vi "StartupGISPollProcess.vi"(8 "error in (no error)":errorcluster, 10 "GIS Printer":refnum<class "GIS Printer.lvclass">, 11 "TopLevel in":refnum<class "TopLevel.lvclass">) -> (0 "error out":errorcluster)   [LabVIEW 2022 SP3, in "GIS Printer.lvclass"]
uses:
  GIS Printer.lvclass
  TopLevel/TopLevel.lvclass
  GIS Poll Process.vi
  GIS Head Poll Process.vi
panel:
  out "Array 2":bool[](array[boolean])
  out "Array":bool[](array[boolean])
  out "timed out?":bool
  out "sync from process?":bool
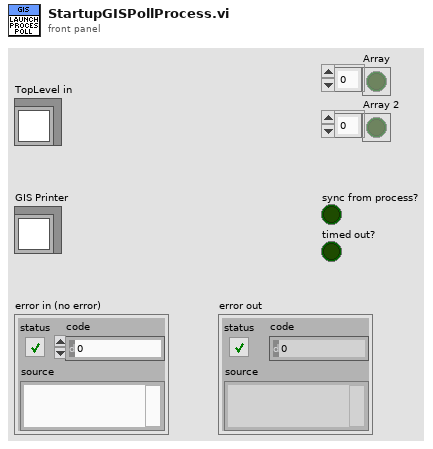
[diagram p1: front panel]
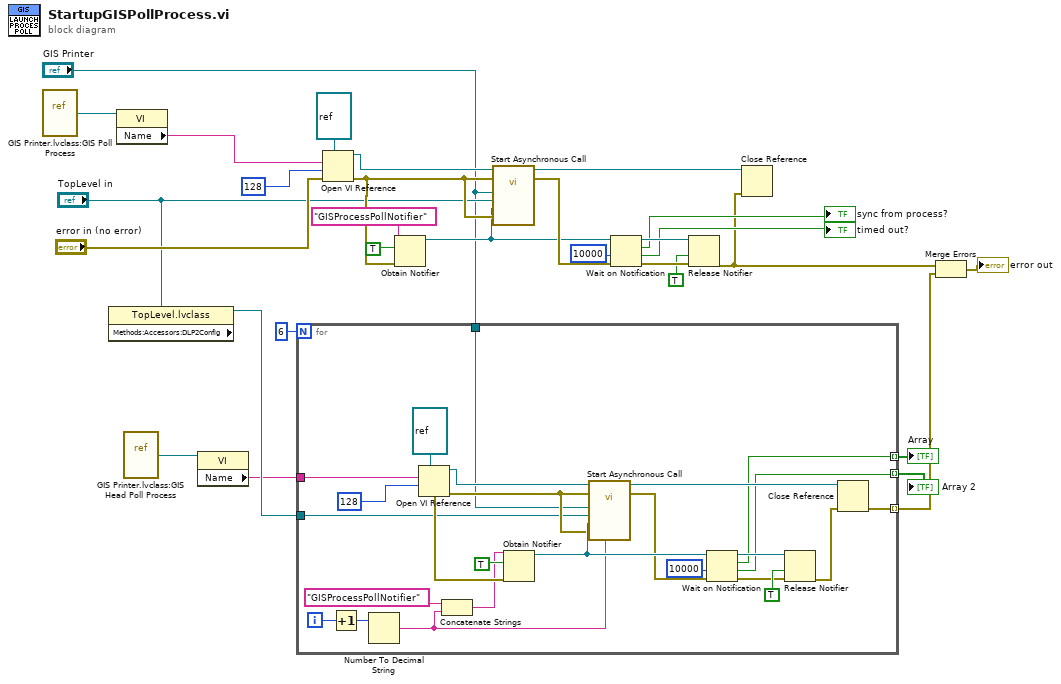
[diagram p0: block diagram]
diagram:
  n1 = vi-ref "GIS Printer.lvclass:GIS Poll Process.vi"() -> (w23:refnum<vi>)
  n2 = property class="TopLevel.lvclass" props=["Methods:Accessors:DLP2Config"](reference="TopLevel in") -> (reference out=w8:refnum<class "TopLevel.lvclass">)  [unwired: 1 in, 2 out]
  n3 = property class="VI"(reference=w23) -> ("Name"=w24:string)  [unwired: 1 in, 2 out]
  n4 = vi-ref "GIS Printer.lvclass:GIS Head Poll Process.vi"() -> (w9:refnum<vi>)
  n5 = property class="VI"(reference=w9) -> ("Name"=w6:string)  [unwired: 1 in, 2 out]
  n6 = for {
    N: 6 -> [_]
    tunnel: w8 -> [w37]
    tunnel: "GIS Printer" -> [w36]
    tunnel: w6 -> [w35]
    tunnel: [w34] -> w2 mode=indexing
    tunnel: [w33] -> w1 mode=indexing
    tunnel: [w31] -> w3 mode=indexing
    i -> [w40]
    n7 = Increment(x=w40) -> (x+1=w32:i32)
    n8 = Number To Decimal String(number=w32) -> (decimal integer string=w30:string)  [unwired: 1 in]
    n9 = Open VI Reference(type specifier VI Refnum (for type only)=refnum<vi> refnum, vi path=w35, options=128) -> (vi reference=w43:refnum<vi>, error out=w46:errorcluster)  [unwired: 3 in]
    n10 = Concatenate Strings("GISProcessPollNotifier" ("name (unnamed)"), w30) -> (w38:string)
    n11 = Obtain Notifier(name (unnamed)=w38, notification data type=TRUE, error in (no error)=w46) -> (notifier out=w53:refnum<notifier>)  [unwired: 1 in, 2 out]
    n12 = call-by-ref "Start Asynchronous Call"(reference=w43, error in=w46, "HeadNo"=w30, 8:"error in (no error)"=w46, "notifierSync"=w53, "TopLevel"=w37, "GIS Printer in"=w36) -> (reference out=w42:refnum<vi>, error out=w51:errorcluster)  [unwired: 5 in, 2 out]
    n13 = Wait on Notification(notifier=w53, timeout in ms (-1)=10000, error in (no error)=w51) -> (notifier out=w49:refnum<notifier>, notification=w34:bool, timed out?=w33:bool, error out=w48:errorcluster)  [unwired: 1 in]
    n14 = Release Notifier(notifier=w49, force destroy? (F)=TRUE, error in (no error)=w48) -> (error out=w52:errorcluster)  [unwired: 2 out]
    n15 = Close Reference(reference=w42, error in (no error)=w52) -> (error out=w31:errorcluster)
  }
  "Array" <- w2
  "Array 2" <- w1
  n16 = Open VI Reference(type specifier VI Refnum (for type only)=refnum<vi> refnum, vi path=w24, options=128, error in (no error)="error in (no error)") -> (vi reference=w26:refnum<vi>, error out=w20:errorcluster)  [unwired: 2 in]
  n17 = Obtain Notifier(name (unnamed)="GISProcessPollNotifier", notification data type=TRUE, error in (no error)=w20) -> (notifier out=w11:refnum<notifier>)  [unwired: 1 in, 2 out]
  n18 = call-by-ref "Start Asynchronous Call"(reference=w26, error in=w20, 8:"error in (no error)"=w20, "notifierSync"=w11, "TopLevel"="TopLevel in", "GIS Printer in"="GIS Printer") -> (reference out=w27:refnum<vi>, error out=w13:errorcluster)  [unwired: 6 in, 2 out]
  n19 = Wait on Notification(notifier=w11, timeout in ms (-1)=10000, error in (no error)=w13) -> (notifier out=w17:refnum<notifier>, notification=→"sync from process?":bool, timed out?=→"timed out?":bool, error out=w18:errorcluster)  [unwired: 1 in]
  n20 = Release Notifier(notifier=w17, force destroy? (F)=TRUE, error in (no error)=w18) -> (error out=w12:errorcluster)  [unwired: 2 out]
  n21 = Close Reference(reference=w27, error in (no error)=w12) -> ()  [unwired: 1 out]
  n22 = Merge Errors(w12, w3) -> (→"error out":errorcluster)
